vi "Proceed.vi"(7 "component is ready (Y)":bool=TRUE, 8 "error in (no error)":errorcluster, 10 "ProceedMessage":refnum<class "ProceedMessage.lvclass">, 11 "Autofocus in":refnum<class "Autofocus.lvclass">) -> (0 "error out":errorcluster, 2 "all observers are ready?":bool, 3 "Autofocus out":refnum<class "Autofocus.lvclass">)   [LabVIEW 2012, in "Autofocus.lvclass"]
doc: "The Proceed method is used to check if your component is ready. Also it checks if the observers are ready. When the observers and the component are ready, it sends the proceed to its observee. If it's the highest observee, it distributes a stop command."
uses:
  Autofocus.lvclass
  <vilib>/Distrio/Murmex/ProceedMessage/ProceedMessage.lvclass
  Autofocus.lvclass/Autofocus.ctl
  <vilib>/Distrio/Murmex/GenericMessage/GenericMessage.lvclass
  <vilib>/Distrio/Murmex/Murmex/Murmex.lvclass
  <vilib>/Distrio/Murmex/Message/Add or replace parameter.vi
  <vilib>/Distrio/Murmex/Message/Message.lvclass
panel:
  # "This method is called when the PROCEED\ntrigger is sent. \n\nOverride this method when your component needs to\nrespond to this trigger. \n\nCall parent for proper implementation"
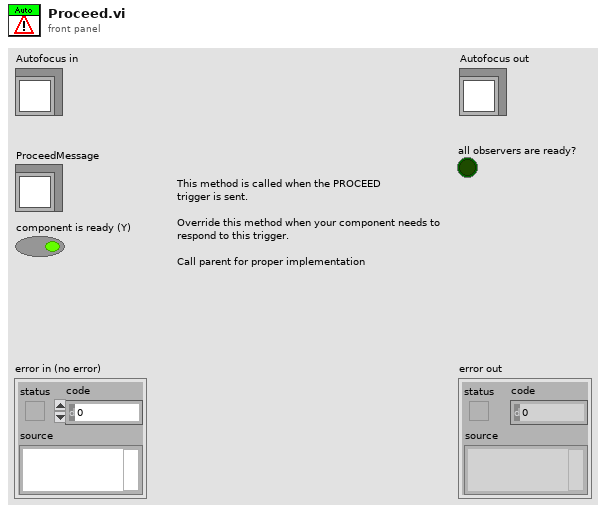
[diagram p1: front panel]
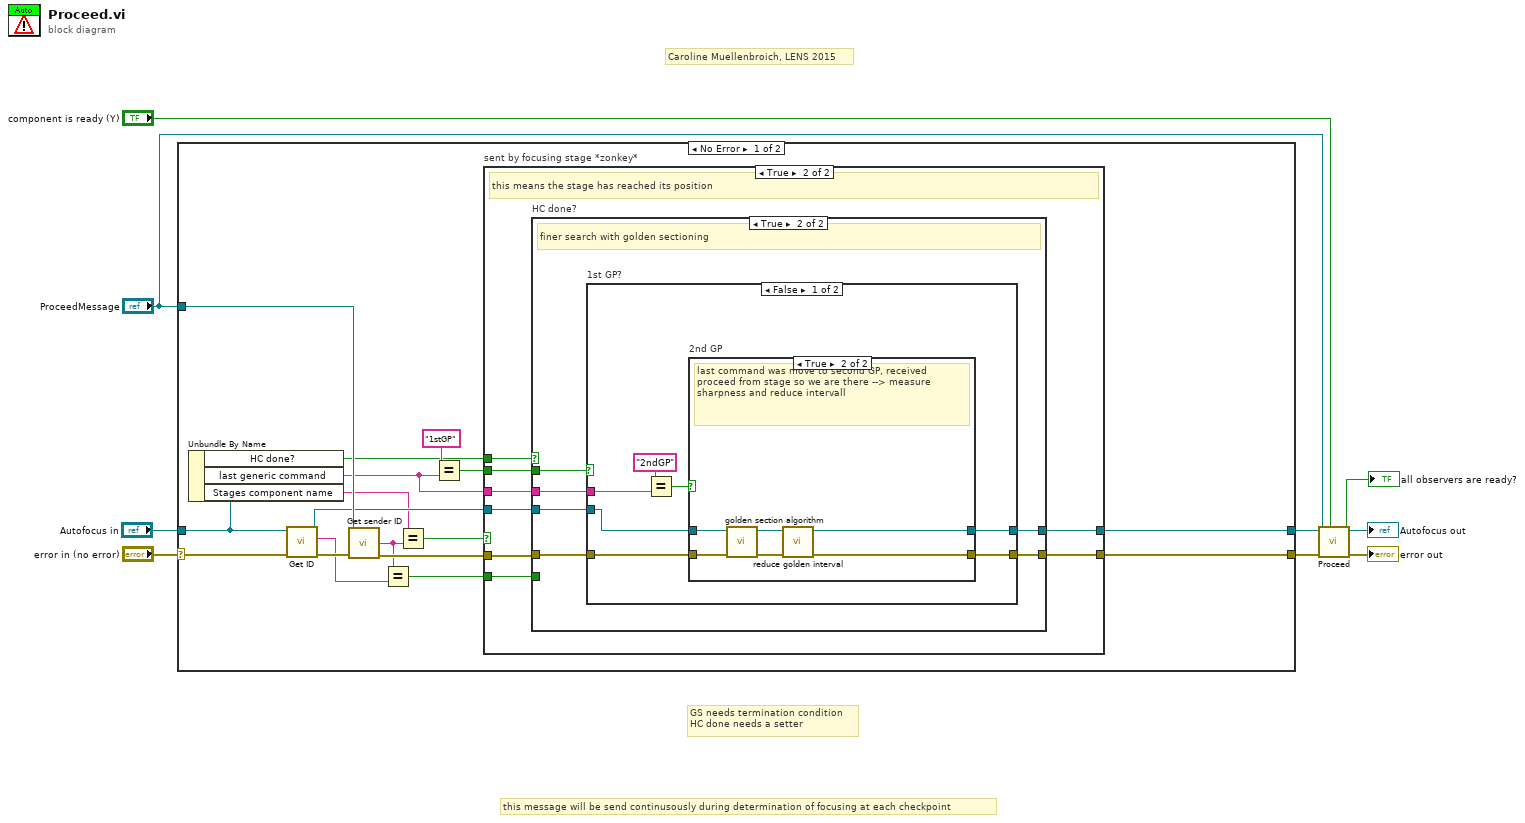
[diagram p0: block diagram]
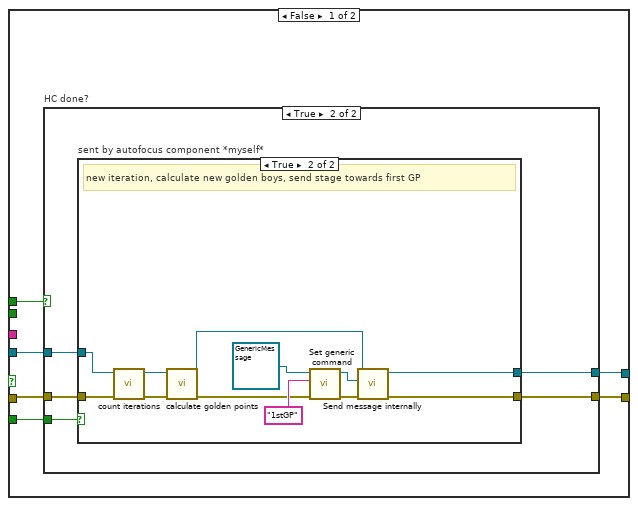
[diagram p2: hidden frame]
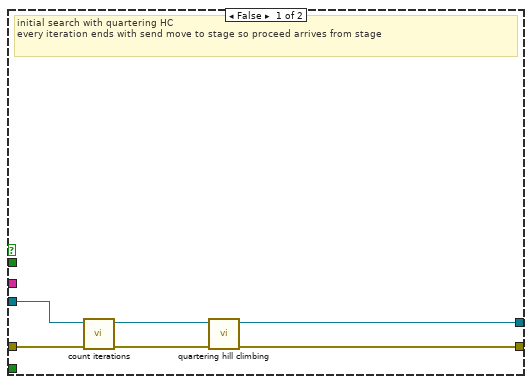
[diagram p5: hidden frame]
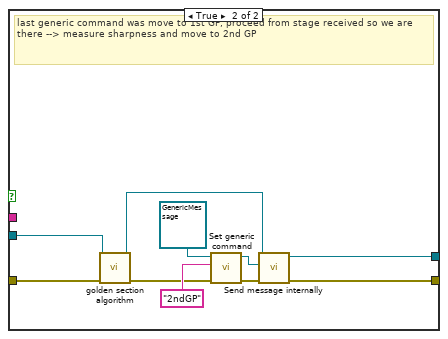
[diagram p7: hidden frame]
diagram:
  # "this message will be send continusously during determination of focusing at each checkpoint"
  # "GS needs termination condition\nHC done needs a setter"
  # "Caroline Muellenbroich, LENS 2015"
  n1 = case shown="No Error" "error in (no error)" {
    selector: "error in (no error)" -> [w11 w100]
    tunnel: [w26 w100] -> w4
    tunnel: "Autofocus in" -> [w10 w99]
    tunnel: [w25 w99] -> w2
    tunnel: "ProceedMessage" -> [w23 _]
    frame No Error {
      n2 = Unbundle By Name(w10) -> ("HC done?"=w13:bool, "last generic command"=w15:string, "Stages component name"=w12:string)
      n3 = call <vilib>:"Get ID.vi"("error in (no error)"=w11, "Murmex in"=w10) -> ("error out"=w22:errorcluster, "component id"=w19:string, "Murmex out"=w14:refnum<class "Autofocus.lvclass">)  [unwired: 7 in]
      n4 = call <vilib>:"Get sender ID.vi"("error in (no error)"=w22, "Message in"=w23) -> ("error out"=w24:errorcluster, "sender"=w20:string)  [unwired: 7 in, 1 out]
      n5 = Equal?(x=w20, y=w19) -> (x = y?=w18:bool)
      n6 = Equal?(x=w12, y=w20) -> (x = y?=w21:bool)
      n7 = Equal?(x="1stGP", y=w15) -> (x = y?=w16:bool)
      n8 = case "sent by focusing stage *zonkey*" shown="True" w21 {
        tunnel: [w29 w61] -> w26
        tunnel: [w27 w60] -> w25
        tunnel: w13 -> [w32 w59]
        tunnel: w24 -> [w30 w58]
        tunnel: w14 -> [w28 w57]
        tunnel: w18 -> [w31 w56]
        tunnel: w16 -> [_ w55]
        tunnel: w15 -> [_ w54]
        frame False {
          n9 = case "HC done?" shown="True" w32 {
            tunnel: w31 -> [_ w39]
            tunnel: w30 -> [w34 w38]
            tunnel: [w34 w37] -> w29
            tunnel: w28 -> [w33 w36]
            tunnel: [w33 w35] -> w27
            frame False {
              # "not sure what happens in this case? not sure if autofocus sends proceed to itself?"
            }
            frame True {
              n10 = case "sent by autofocus component *myself*" shown="True" w39 {
                tunnel: w38 -> [w41 w45]
                tunnel: [w41 w47] -> w37
                tunnel: w36 -> [w40 w43]
                tunnel: [w40 w46] -> w35
                frame False {
                }
                frame True {
                  # "new iteration, calculate new golden boys, send stage towards first GP"
                  n11 = call-dynamic "count iterations.vi"("error in (no error)"=w45, "Autofocus in"=w43) -> ("error out"=w44:errorcluster, "Autofocus out"=w42:refnum<class "Autofocus.lvclass">)  [unwired: 8 in]
                  n12 = call-dynamic "calculate golden points.vi"("error in (no error)"=w44, "Autofocus in"=w42) -> ("error out"=w49:errorcluster, "Autofocus out"=w48:refnum<class "Autofocus.lvclass">)  [unwired: 6 in, 2 out]
                  n13 = call <vilib>:"Set generic command.vi"("error in (no error)"=w49, "generic command"="1stGP", "GenericMessage in"=refnum<class "GenericMessage.lvclass"> refnum ("Distrio Murmex 1.2:GenericMessage")) -> ("error out"=w51:errorcluster, "GenericMessage out"=w50:refnum<class "GenericMessage.lvclass">)  [unwired: 7 in]
                  n14 = call <vilib>:"Send message internally.vi"("error in (no error)"=w51, "Message"=w50, "Murmex in"=w48) -> ("error out"=w47:errorcluster, "Murmex out"=w46:refnum<class "Autofocus.lvclass">)  [unwired: 7 in]
                }
              }
            }
          }
        }
        frame True {
          # "this means the stage has reached its position"
          n15 = case "HC done?" shown="True" w59 {
            tunnel: w58 -> [w65 w73]
            tunnel: [w67 w72] -> w61
            tunnel: w57 -> [w64 w71]
            tunnel: [w66 w70] -> w60
            tunnel: w56 -> [_ _]
            tunnel: w55 -> [_ w69]
            tunnel: w54 -> [_ w68]
            frame False {
              # "initial search with quartering HC\nevery iteration ends with send move to stage so proceed arrives from stage"
              n16 = call-dynamic "count iterations.vi"("error in (no error)"=w65, "Autofocus in"=w64) -> ("error out"=w62:errorcluster, "Autofocus out"=w63:refnum<class "Autofocus.lvclass">)  [unwired: 8 in]
              n17 = call-dynamic "quartering hill climbing.vi"("error in (no error)"=w62, "Autofocus in"=w63) -> ("error out"=w67:errorcluster, "Autofocus out"=w66:refnum<class "Autofocus.lvclass">)  [unwired: 8 in]
            }
            frame True {
              # "finer search with golden sectioning"
              n18 = case "1st GP?" shown="False" w69 {
                tunnel: w73 -> [w77 w92]
                tunnel: [w76 w98] -> w72
                tunnel: w71 -> [w75 w90]
                tunnel: [w74 w93] -> w70
                tunnel: w68 -> [w78 _]
                frame False {
                  n19 = Equal?(x="2ndGP", y=w78) -> (x = y?=w79:bool)
                  n20 = case "2nd GP" shown="True" w79 {
                    tunnel: w77 -> [w81 w88]
                    tunnel: [w81 w86] -> w76
                    tunnel: w75 -> [w82 w85]
                    tunnel: [w82 w83] -> w74
                    frame False {
                    }
                    frame True {
                      # "last command was move to second GP, received proceed from stage so we are there --> measure sharpness and reduce intervall"
                      n21 = call-dynamic "golden section algorithm.vi"("error in (no error)"=w88, "Autofocus in"=w85) -> ("error out"=w87:errorcluster, "Autofocus out"=w84:refnum<class "Autofocus.lvclass">)  [unwired: 8 in]
                      n22 = call-dynamic "reduce golden interval.vi"("error in (no error)"=w87, "Autofocus in"=w84) -> ("error out"=w86:errorcluster, "Autofocus out"=w83:refnum<class "Autofocus.lvclass">)  [unwired: 8 in]
                    }
                  }
                }
                frame True {
                  # "last generic command was move to 1st GP, proceed from stage received so we are there --> measure sharpness and move to 2nd GP"
                  n23 = call-dynamic "golden section algorithm.vi"("error in (no error)"=w92, "Autofocus in"=w90) -> ("error out"=w91:errorcluster, "Autofocus out"=w89:refnum<class "Autofocus.lvclass">)  [unwired: 8 in]
                  n24 = call <vilib>:"Set generic command.vi"("error in (no error)"=w91, "generic command"="2ndGP", "GenericMessage in"=refnum<class "GenericMessage.lvclass"> refnum ("Distrio Murmex 1.2:GenericMessage")) -> ("error out"=w95:errorcluster, "GenericMessage out"=w94:refnum<class "GenericMessage.lvclass">)  [unwired: 7 in]
                  n25 = call <vilib>:"Send message internally.vi"("error in (no error)"=w95, "Message"=w94, "Murmex in"=w89) -> ("error out"=w98:errorcluster, "Murmex out"=w93:refnum<class "Autofocus.lvclass">)  [unwired: 7 in]
                }
              }
            }
          }
        }
      }
    }
    frame Error {
    }
  }
  n26 = call-parent "Proceed.vi"("component is ready (Y)"="component is ready (Y)", "error in (no error)"=w4, "ProceedMessage"="ProceedMessage", "Murmex in"=w2) -> ("error out"=→"error out":errorcluster, "all observers are ready?"=→"all observers are ready?":bool, "Murmex out"=→"Autofocus out":refnum<class "Autofocus.lvclass">)  [unwired: 5 in]
